vi "Pre Launch Init.vi"(11 "DAQ in":refnum<class "DAQ.lvclass">) -> (0 "error out":errorcluster, 3 "DAQ out":refnum<class "DAQ.lvclass">)   [LabVIEW 2011, in "DAQ.lvclass"]
doc: "(<B>Filename</B>: Actor Framework.lvlib:Actor.lvclass:Pre Launch Init.vi)\n\nDefines behavior that occurs after the Launch Actor method is invoked but before the actor's Actor Core method begins running.\n\nThe Pre Launch Init method is guaranteed to finish before the Launch Actor method returns to its caller and before the actor itself receives any messages. Any references that the Pre Launch Init method obtains are guaranteed to have the same lifetime as the actor itself. Any errors that the Pre Launch Init method returns will abort the launch.\n\nBy default, this method does nothing. A descendant class may override it to define behavior."
uses:
  DAQ.lvclass
  <vilib>/LabVIEW Interface for Arduino/LabVIEW Interface for Arduino.lvlib
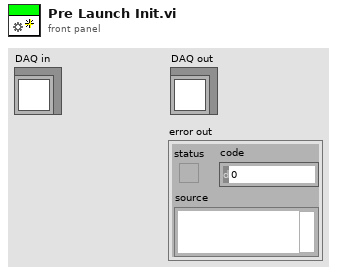
[diagram p1: front panel]
types:
  T1 = typedef "LabVIEW Interface for Arduino.lvlib/Arduino Resource.ctl" = cluster{"VISA resource":refnum<visa-resource-name>, "Board Type":T2, "Connection Type":enum8{"USB / Serial"}, "Bytes Per Packet (15)":u8}
  T2 = typedef "LabVIEW Interface for Arduino.lvlib/Board Type.ctl" = enum16{"Uno", "Dimuelanove w/Atmega 328", "Mega 2560"}
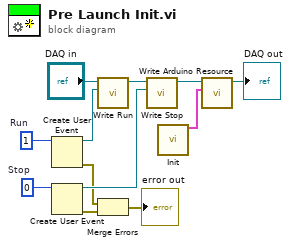
[diagram p0: block diagram]
diagram:
  w11 = 0  # Stop
  w12 = 1  # Run
  n1 = Create User Event(user event datatype=w12) -> (user event=w10:refnum<user-event>, error out=w5:errorcluster)  [unwired: 1 in]
  n2 = Create User Event(user event datatype=w11) -> (user event=w7:refnum<user-event>, error out=w4:errorcluster)  [unwired: 1 in]
  n3 = call "Write Run.vi"("Run"=w10, "DAQ in"="DAQ in") -> ("DAQ out"=w8:refnum<class "DAQ.lvclass">)  [unwired: 9 in]
  n4 = Merge Errors(w5, w4) -> (→"error out":errorcluster)
  n5 = call "Write Stop.vi"("Stop"=w7, "DAQ in"=w8) -> ("DAQ out"=w2:refnum<class "DAQ.lvclass">)  [unwired: 9 in]
  n6 = call <vilib>:"Init.vi"() -> ("Arduino Resource"=w3:T1)  [unwired: 18 in, 1 out]
  n7 = call "Write Arduino Resource.vi"("Arduino Resource"=w3, "DAQ in"=w2) -> ("DAQ out"=→"DAQ out":refnum<class "DAQ.lvclass">)  [unwired: 9 in]
